vi "LX-ReadGlobaRadioParams.vi"(8 "error in (no error)":errorcluster caption="错误输入（无错误）", 11 "名称或相对路径":string="Template Program") -> (0 "错误输出":errorcluster, 2 "ParamsUI":T1={"IsNorImage"=TRUE, "Exposure Values"=100289, "ImagePath"=path "C:/Users/hedongpo/Desktop/514-hdp/Alignment Assemble System/Test Picture/B/3.bmp"}, 3 "ParamsUI 内圆":T5={"圆参数1"={"Search  Direction"=0, "Edge Options"={"Edge Polarity"=0, "Kernel Size"=3, "Width"=3, "Minimum Edge Strength"=50.0, "Interpolation Type"=enum."Bilinear Fixed", "Data Processing Method"=enum."Average"}, "Show Search Area"=TRUE, "Show Search Lines"=TRUE, "Show Edges Found"=TRUE, "Show Result"=TRUE, "Search Area Color"=65280, "Search Lines Color"=255, "Edge Locations Color"=16776960, "Result Color"=16711680, "Overlay Group Name"=""}, "圆参数"={"Process"=enum."Get First Edge", "Step Size"=1, "Max Pixel Radius"=3}, "圆环ROI设定"={"Center X"=1717, "Center Y"=1486, "Inner Radius"=327, "Outer Radius"=1645, "Start Angle"=0.0, "End Angle"=0.0}, "Show Search Area"=TRUE, "Show Search Lines"=TRUE, "Show Edges Found"=TRUE, "Show Result"=TRUE, "200次模板表格"=path "C:/Users/Administrator/Desktop/GRR模板/Test.xlsx", "GRR模板表格"=path "C:/Users/Administrator/Desktop/GRR模板/Test.xlsx", "孔径规格"={"孔径上限"="0.014", "孔径标准值"="1.1", "孔径下限"="0"}} {"圆参数1"."Search  Direction" items=["Outside to Inside", "Inside to Outside"]; "圆参数1"."Edge Options"."Edge Polarity" items=["All Edges", "Rising Edges", "Falling Edges"]; "圆参数1"."Edge Options"."Minimum Edge Strength" format="%.2f"; "圆参数1"."Edge Options"."Width" step=2; "圆参数1"."Edge Options"."Kernel Size" step=2; "圆环ROI设定"."End Angle" min=-90.0 max=90.0 step=1.0 format="%.2f"; "圆环ROI设定"."Start Angle" min=-90.0 max=90.0 step=1.0 format="%.2f"; "圆环ROI设定"."Center X" scale=0.0..1024.0})   [LabVIEW 2017]
uses:
  <vilib>/vision/Measure.llb/Edge Options.ctl
  <vilib>/vision/Measure.llb/Edge Polarity.ctl
  Global System.vi
  <vilib>/Utility/xml.llb/Read From XML File(string).vi
panel:
  out "添加的路径":path
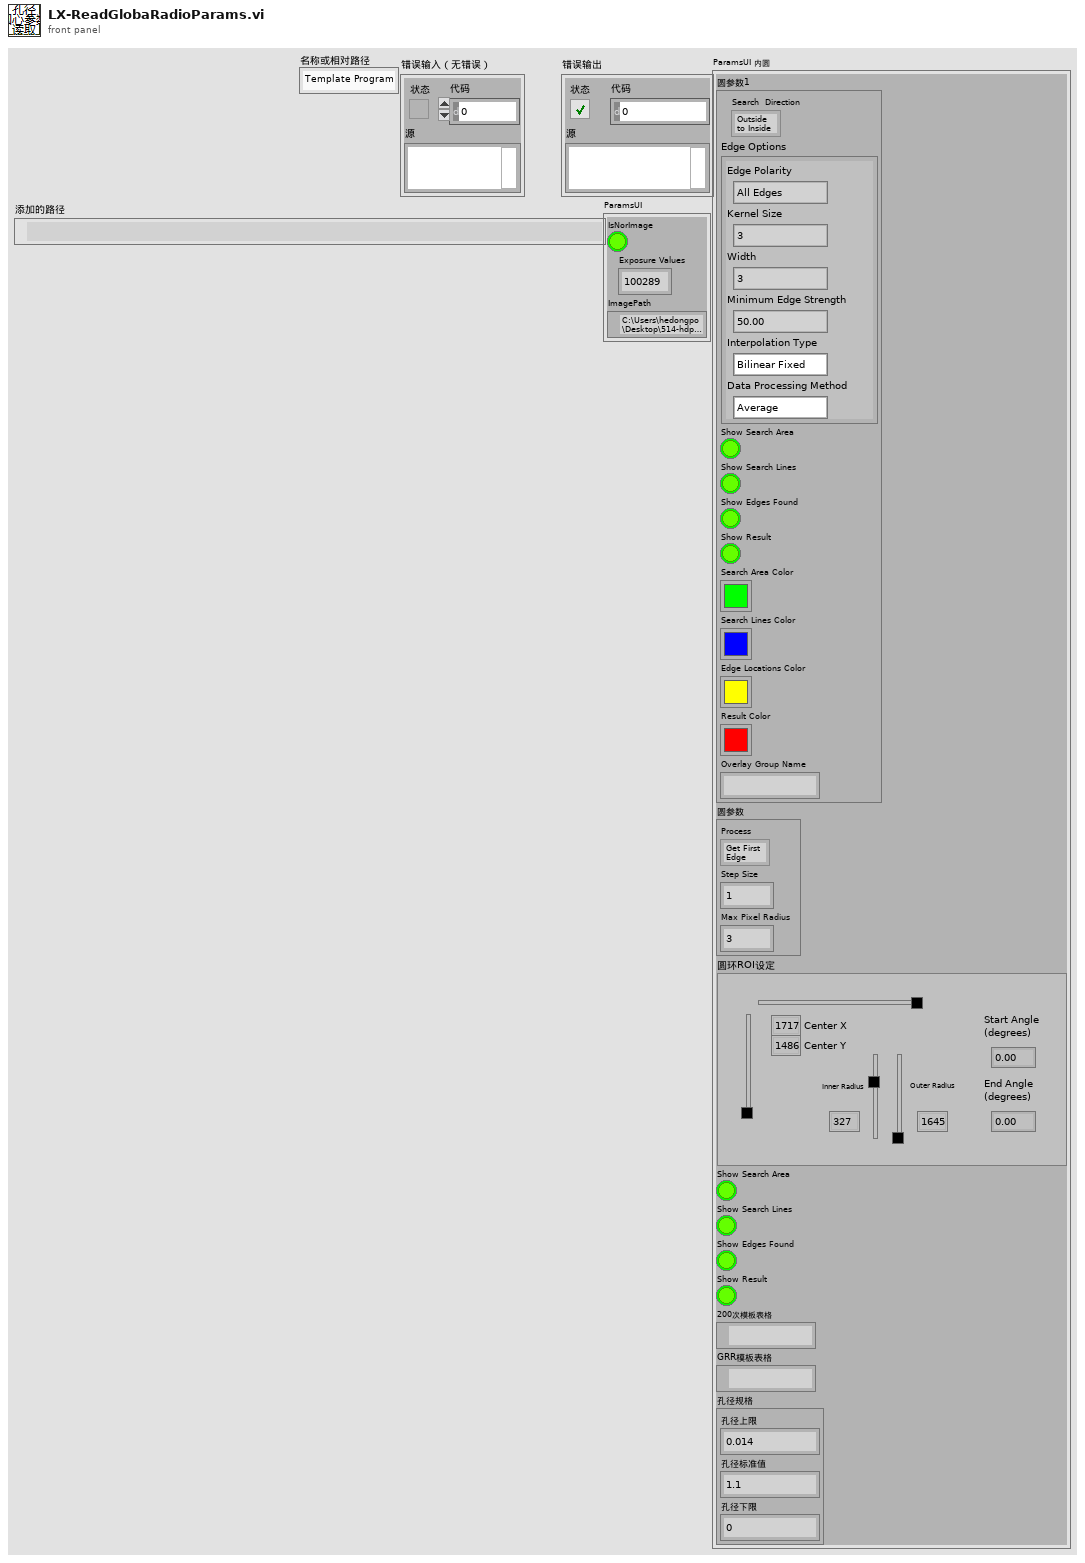
[diagram p1: front panel]
types:
  T1 = cluster{"IsNorImage":bool, "Exposure Values":u32, "ImagePath":path}
  T2 = typedef "Edge Options.ctl" = cluster{"Edge Polarity":T3, "Kernel Size":u32, "Width":u32, "Minimum Edge Strength":sgl, "Interpolation Type":enum32{"Zero Order", "Bilinear", "Quadratic", "Cubic", "Bilinear Fixed"}, "Data Processing Method":enum32{"Average", "Median"}}
  T3 = typedef "Edge Polarity.ctl" = u32
  T4 = typedef "IMAQ Circle" = cluster{"Center X":i32, "Center Y":i32, "Inner Radius":i32, "Outer Radius":i32, "Start Angle":dbl, "End Angle":dbl}
  T5 = cluster{"圆参数1":cluster{"Search  Direction":u32, "Edge Options":T2, "Show Search Area":bool, "Show Search Lines":bool, "Show Edges Found":bool, "Show Result":bool, "Search Area Color":u32, "Search Lines Color":u32, "Edge Locations Color":u32, "Result Color":u32, "Overlay Group Name":string}, "圆参数":cluster{"Process":enum16{"Get First Edge", "Get First + Last Edge", "Get All Edges", "Get Best Edge"}, "Step Size":i32, "Max Pixel Radius":i32}, "圆环ROI设定":T4, "Show Search Area":bool, "Show Search Lines":bool, "Show Edges Found":bool, "Show Result":bool, "200次模板表格":path, "GRR模板表格":path, "孔径规格":cluster{"孔径上限":string, "孔径标准值":string, "孔径下限":string}}
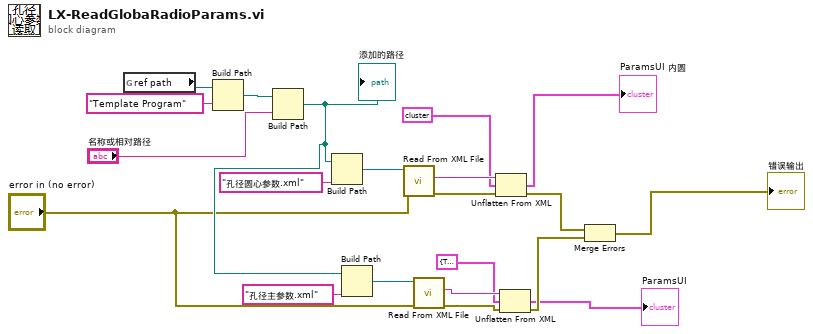
[diagram p0: block diagram]
diagram:
  n1 = global read "Global System.vi" "ref path"() -> (w17:path)
  n2 = Build Path(base path=w17, name or relative path="Template Program" ("名称或相对路径")) -> (appended path=w15:path)
  n3 = Build Path(base path=w15, name or relative path="名称或相对路径") -> (appended path=w9:path)
  "添加的路径" <- w9
  n4 = Build Path(base path=w9, name or relative path="孔径圆心参数.xml" ("名称或相对路径")) -> (appended path=w20:path)
  n5 = Build Path(base path=w9, name or relative path="孔径主参数.xml" ("名称或相对路径")) -> (appended path=w10:path)
  n6 = call-poly <vilib>:"Read From XML File.vi"("error in (no error)"="error in (no error)", "XML File Path"=w20) -> ("error out"=w14:errorcluster, "XML Elements"=w21:string)  [unwired: 7 in, 1 out]
  n7 = call-poly <vilib>:"Read From XML File.vi"("error in (no error)"="error in (no error)", "XML File Path"=w10) -> ("error out"=w6:errorcluster, "XML Elements"=w7:string)  [unwired: 7 in, 1 out]
  n8 = Unflatten From XML(xml string=w21, type=T5 {"圆参数1"={"Search  Direction"=0, "Edge Options"={"Edge Polarity"=0, "Kernel Size"=3, "Width"=3, "Minimum Edge Strength"=50.0, "Interpolation Type"=enum."Bilinear Fixed", "Data Processing Method"=enum."Average"}, "Show Search Area"=TRUE, "Show Search Lines"=TRUE, "Show Edges Found"=TRUE, "Show Result"=TRUE, "Search Area Color"=65280, "Search Lines Color"=255, "Edge Locations Color"=16776960, "Result Color"=16711680, "Overlay Group Name"=""}, "圆参数"={"Process"=enum."Get First Edge", "Step Size"=1, "Max Pixel Radius"=3}, "圆环ROI设定"={"Center X"=1717, "Center Y"=1486, "Inner Radius"=327, "Outer Radius"=1645, "Start Angle"=0.0, "End Angle"=0.0}, "Show Search Area"=TRUE, "Show Search Lines"=TRUE, "Show Edges Found"=TRUE, "Show Result"=TRUE, "200次模板表格"=path "C:/Users/Administrator/Desktop/GRR模板/Test.xlsx", "GRR模板表格"=path "C:/Users/Administrator/Desktop/GRR模板/Test.xlsx", "孔径规格"={"孔径上限"="0.014", "孔径标准值"="1.1", "孔径下限"="0"}} ("ParamsUI 内圆"), error in (no error)=w14) -> (value=→"ParamsUI 内圆":T5, error out=w4:errorcluster)
  n9 = Unflatten From XML(xml string=w7, type=T1 {"IsNorImage"=TRUE, "Exposure Values"=100289, "ImagePath"=path "C:/Users/hedongpo/Desktop/514-hdp/Alignment Assemble System/Test Picture/B/3.bmp"} ("ParamsUI"), error in (no error)=w6) -> (value=→"ParamsUI":T1, error out=w5:errorcluster)
  n10 = Merge Errors(w4, w5) -> (→"错误输出":errorcluster)
